vi "Init Messaging.vi"(8 "error in (no error)":errorcluster, 11 "LV Client in":refnum<class "LV Client.lvclass">) -> (0 "error out":errorcluster, 3 "LV Client out":refnum<class "LV Client.lvclass">)   [LabVIEW 2020, in "LV Client.lvclass"]
uses:
  LV Client.lvclass
  LV Client.lvclass/LV Client.ctl
  Connection State Callback.vi
  Message Callback.vi
  <vilib>/IlluminatedG/lv-msg-simple/Stream-Simple-Msg/Manager/Manager.lvclass
  Common/Message ID.ctl
  Common/Common.lvlib
  3b13d6b0-30b0-4344-bcb4-468328f35f02.vi
  <vilib>/IlluminatedG/lv-stream-tcp/Stream-TCP.lvlib
  <vilib>/IlluminatedG/lv-stream/Endpoint/Endpoint.lvclass
  <vilib>/IlluminatedG/lv-stream-tcp/TCP Client/TCP Client.lvclass
  C:/Program Files (x86)/National Instruments/LabVIEW 2020/vi.lib/IlluminatedG/lv-stream/Connection/Connection.lvclass
  C:/Program Files (x86)/National Instruments/LabVIEW 2020/vi.lib/IlluminatedG/lv-stream/Endpoint/Endpoint.lvclass
  C:/Program Files (x86)/National Instruments/LabVIEW 2020/vi.lib/IlluminatedG/lv-stream-tcp/TCP Client/TCP Client.lvclass
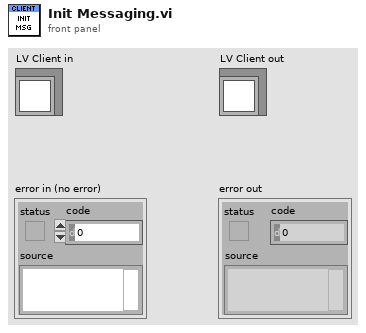
[diagram p1: front panel]
types:
  T1 = typedef "Common.lvlib/Message ID.ctl" = enum16{"Timer State", "Timer Value", "Timer Start", "Timer Pause", "Timer Reset", "Timer Init"}
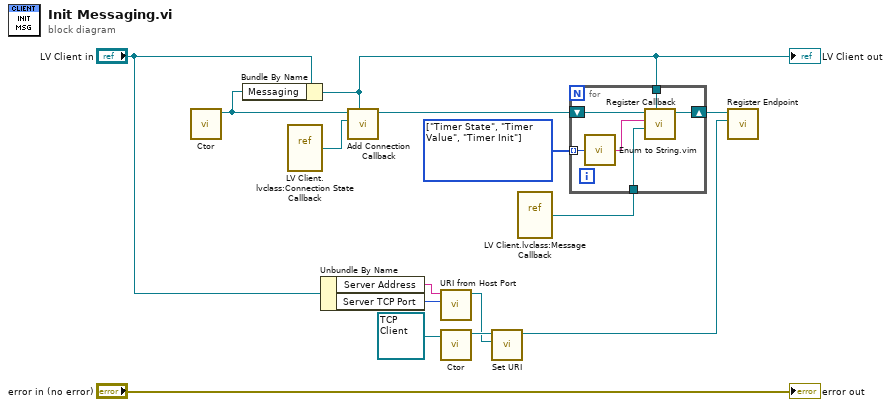
[diagram p0: block diagram]
diagram:
  w14 = T1[] [enum."Timer State", enum."Timer Value", enum."Timer Init"] items=["Timer State", "Timer Value", "Timer Start", "Timer Pause", "Timer Reset", "Timer Init"]
  n1 = call <vilib>:"Ctor.vi"() -> ("Manager out"=w13:refnum<class "Manager.lvclass">)  [unwired: 10 in, 1 out]
  n2 = Bundle By Name(cluster="LV Client in", "Messaging"=w13) -> (w12:refnum<class "LV Client.lvclass">)
  "LV Client out" <- w12
  n3 = vi-ref "LV Client.lvclass:Connection State Callback.vi"() -> (w11:refnum<vi>)
  n4 = Unbundle By Name("LV Client in") -> ("Server Address"=w6:string, "Server TCP Port"=w5:u16)
  n5 = call <vilib>:"Add Connection Callback.vi"("Owner"=w12, "Callback"=w11, "Manager in"=w13) -> ("Manager out"=w10:refnum<class "Manager.lvclass">)  [unwired: 7 in, 1 out]
  n6 = call <vilib>:"URI from Host Port.vi"("Port"=w5, "Host"=w6) -> ("URI"=w3:refnum<class "URI.lvclass">)  [unwired: 9 in]
  n7 = call-dynamic <vilib>:"Ctor.vi"("TCP Client in"=refnum<class "TCP Client.lvclass"> refnum) -> ("TCP Client out"=w4:refnum<class "TCP Client.lvclass">)  [unwired: 9 in, 1 out]
  n8 = call <vilib>:"Set URI.vi"("URI"=w3, "Endpoint in"=w4) -> ("Endpoint out"=w2:refnum<class "TCP Client.lvclass">)  [unwired: 8 in, 1 out]
  n9 = vi-ref "LV Client.lvclass:Message Callback.vi"() -> (w9:refnum<vi>)
  n10 = for {
    tunnel: w12 -> [w20]
    tunnel: w14 -> [w19] mode=indexing
    tunnel: w9 -> [w17]
    shift-right: [w16] -> w8
    shift-left: w10 -> [w21]
    n11 = call "Enum to String.vim"("Enum"=w19) -> ("Enum String"=w18:string)
    n12 = call <vilib>:"Register Callback.vi"("Owner"=w20, "Callback"=w17, "Message ID"=w18, "Manager in"=w21) -> ("Manager out"=w16:refnum<class "Manager.lvclass">)  [unwired: 6 in, 1 out]
  }
  n13 = call <vilib>:"Register Endpoint.vi"("Stream:Endpoint"=w2, "Manager in"=w8) -> ()  [unwired: 8 in, 2 out]
  "error out" <- "error in (no error)"
